vi "TCPRead_Write_GlobalVariables.vi"() -> ()   [LabVIEW 2016]
panel:
  in  "Bytes Written":dbl
  in  "TCP Output":string
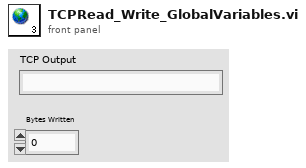
[diagram p1: front panel]
diagram:
